vi "Set Enable State on Multiple Controls.vi"(10 "Disabled":T1(ring), 11 "Controls":refnum<vi>[](array[refnum]) caption="컨트롤") -> ()   [LabVIEW 2018, in "Library-Ctrl.lvlib"]
doc: "입력 배열의 모든 컨트롤을 \"활성화 상태\" 값으로 설정합니다."
uses:
  Library-Ctrl.lvlib
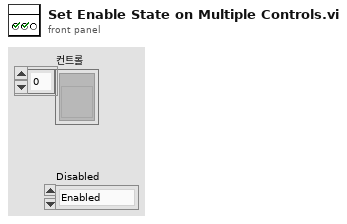
[diagram p1: front panel]
types:
  T1 = enum8{"Enabled", "Disabled", "Disabled and Grayed Out"}
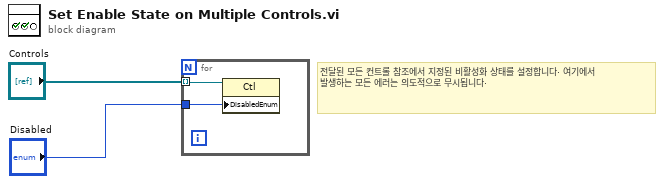
[diagram p0: block diagram]
diagram:
  # "전달된 모든 컨트롤 참조에서 지정된 비활성화 상태를 설정합니다. 여기에서 발생하는 모든 에러는 의도적으로 무시됩니다."
  n1 = for {
    tunnel: "Controls" -> [w4] mode=indexing
    tunnel: "Disabled" -> [w3]
    n2 = property class="Ctl"(reference=w4, "DisabledEnum"=w3) -> ()  [unwired: 1 in, 2 out]
  }
